vi "LIA-Simulator.vi"() -> ()   [LabVIEW 2018]
uses:
  <vilib>/addons/Digital Filter Design/_Objects.llb/DFD Multirate Filter Specification (Design).ctl
  <vilib>/addons/Digital Filter Design/_Objects.llb/DFD Filter Ripple Specification (Design).ctl
  <vilib>/Analysis/4window.llb/windowTd.ctl
  <vilib>/addons/Digital Filter Design/Analysis.llb/DFD Plot Freq Response (Linear-Spaced).vi
  <vilib>/addons/Digital Filter Design/Design.llb/DFD MRate Filter Design (Integer).vi
  <vilib>/addons/Digital Filter Design/Process.llb/DFD Filtering (Array).vi
  <vilib>/Analysis/2dsp.llb/Decimate (continuous, CDB).vi
  <vilib>/addons/Digital Filter Design/Multirate.llb/DFD MRate Filtering for Single Block (Array).vi
  <vilib>/measure/maspectr.llb/FFT Power Spectrum and PSD for 1 Chan (CDB).vi
  <vilib>/measure/maspectr.llb/FFT Power Spectrum and PSD for 1 Chan.vi
  <vilib>/measure/NI_MAPro.lvlib
  <vilib>/Analysis/NI_AALPro.lvlib
  <vilib>/addons/Digital Filter Design/NI_DigFilterLicensed.lvlib
  <vilib>/Analysis/NI_AALBase.lvlib
panel:
  in  "Iterations":i32=10
  out "FFT Gain":dbl
  out "Audio Depth":dbl format="%#_p"
  in  "Resolution":dbl=19.0 format="%#_13g"
  in  "Sampling Rate":dbl=1.0 format="%#_p"
  in  "Number Samples":i32=100000
  out "Error Out":errorcluster
  in  "Error In":errorcluster
  in  "Stop":bool
  in  "Tab Control 3":T1(tab)
  out "Noise vrms":dbl
  out "Noise (W|50ohms)":dbl
  out "k":dbl
  out "standard deviation":dbl format="%0.2p"
  out "mean":dbl format="%0.2p"
  out "standard deviation 2":dbl format="%0.2p"
  out "mean 2":dbl format="%0.2p"
  out "mean 3":dbl format="%0.2p"
  out "standard deviation 3":dbl format="%0.2p"
  in  "Tab Control 2":T2(tab)
  out "Waveform Graph 1":dbl[][](graph)
  out "Waveform Graph 3":cluster{"f0":dbl, "df":dbl, "magnitude":dbl[]}(graph)
  out "Waveform Graph 8":dbl[][](graph)
  out "Waveform Graph 7":cluster{"f0":dbl, "df":dbl, "magnitude":dbl[]}(graph)
  out "Waveform Graph 10":dbl[](graph)
  out "Waveform Graph 9":cluster{"f0":dbl, "df":dbl, "magnitude":dbl[]}(graph)
  out "Waveform Graph 12":dbl[](graph)
  out "Waveform Graph 11":cluster{"f0":dbl, "df":dbl, "magnitude":dbl[]}(graph)
  out "Waveform Graph 14":dbl[][](graph)
  out "Waveform Graph 13":cluster{"f0":dbl, "df":dbl, "magnitude":dbl[]}(graph)
  out "Waveform Graph 17":cluster{"f0":dbl, "df":dbl, "values":dbl[]}[](graph)
  out "Waveform Graph 16":dbl[](graph)
  out "Waveform Graph 15":cluster{"f0":dbl, "df":dbl, "magnitude":dbl[]}(graph)
  out "Waveform Graph 21":cluster{"f0":dbl, "df":dbl, "values":dbl[]}[](graph)
  out "Waveform Graph 23":dbl[](graph)
  out "Waveform Graph 22":cluster{"f0":dbl, "df":dbl, "magnitude":dbl[]}(graph)
  out "Waveform Graph 18":cluster{"f0":dbl, "df":dbl, "values":dbl[]}[](graph)
  out "Waveform Graph 20":dbl[](graph)
  out "Waveform Graph 19":cluster{"f0":dbl, "df":dbl, "magnitude":dbl[]}(graph)
  in  "Tab Control 1":T3(tab)
  in  "Oscillator Frequency":dbl=0.1 format="%#_p"
  in  "Oscillator Magnitude":dbl=1.0 format="%#_13g"
  in  "Signal Frequency":dbl=0.1 format="%#_p"
  in  "Signal Offset":cdb format="%#_13g"
  in  "Singal Amplitude":dbl=1.0 format="%#_13g"
  in  "Desired SNR (dB)":dbl format="%#_p"
  in  "low cutoff freq [Hz] 1":dbl=0.2
  in  "stopband atten [dB] 1":dbl=60.0 format="%.2f"
  in  "Decimation 1":i32=4
  in  "Decimation 2":i32=16
  in  "ripple specs":T4={"passband"=0.1, "stopband"=20.0, "dB/linear? (T: dB)"=TRUE}
  in  "freq specs [Hz]":T5={"fpass"=0.001, "fstop"=0.002}
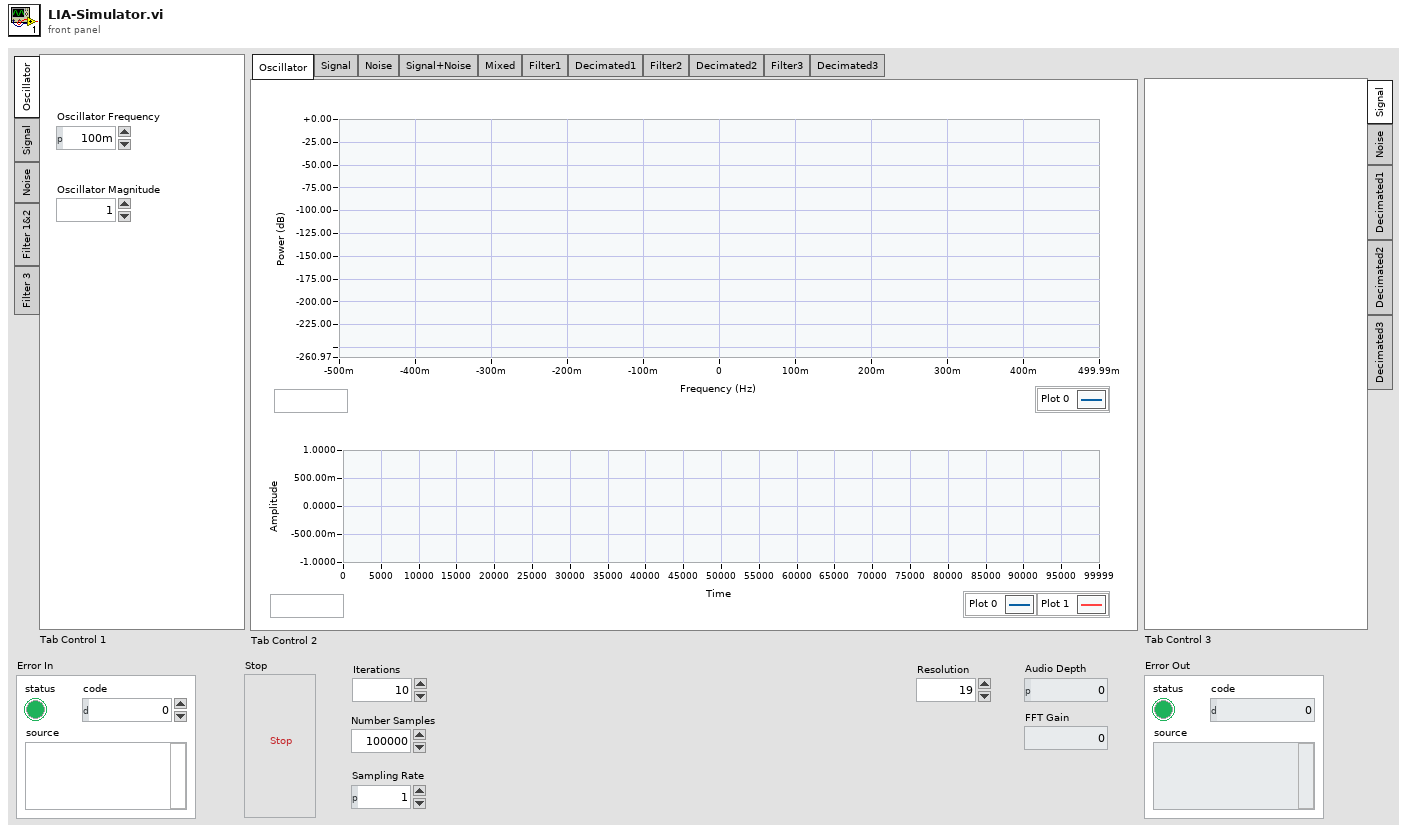
[diagram p1: front panel]
types:
  T1 = enum32{"Signal", "Noise", "Decimated1", "Decimated2", "Decimated3"}
  T2 = enum32{"Oscillator", "Signal", "Noise", "Signal+Noise", "Mixed", "Filter1", "Decimated1", "Filter2", "Decimated2", "Filter3", "Decimated3"}
  T3 = enum32{"Oscillator", "Signal", "Noise", "Filter 1&2", "Filter 3"}
  T4 = typedef "NI_DigFilterLicensed.lvlib/DFD Filter Ripple Specification (Design).ctl" = cluster{"passband":dbl, "stopband":dbl, "dB/linear? (T: dB)":bool}
  T5 = typedef "NI_DigFilterLicensed.lvlib/DFD Multirate Filter Specification (Design).ctl" = cluster{"fpass":dbl, "fstop":dbl}
  T6 = typedef "NI_DigFilterLicensed.lvlib/DFD Filter Obj.ctl" = cluster{"mSRate_Fs":dbl, "mSRate_Version":string, "mSRate_Comments":string, "mSRate_OrgCoef":T7, "mSRate_CurCoef":T7, "mSRate_Quantized?":bool, "mSRate_QCoef":T7, "mSRate_QSettings":T9[], "mSRate_Order":i32, "mSRate_Scaling":cluster{"mSRate_ScaleByPowerOf2?":bool, "mSRate_ScaleType":T11}}
  T7 = typedef "NI_DigFilterLicensed.lvlib/DFD Filter Coef.ctl" = cluster{"type":T8, "gain":dbl, "coef a (k)":dbl[], "coef b (v)":dbl[]}
  T8 = typedef "NI_DigFilterLicensed.lvlib/DFD Filter Structure Type Selector.ctl" = enum16{"Undefined", "FIR Direct Form", "FIR Direct Form Transposed", "FIR Symmetric", "FIR Antisymmetric", "IIR Direct Form I", "IIR Direct Form I Transposed", "IIR Direct Form II", "IIR Direct Form II Transposed", "IIR Cascaded Second Order Sections Form I", "IIR Cascaded Second Order Sections Form I Transposed", "IIR Cascaded Second Order Sections Form II", "IIR Cascaded Second Order Sections Form II Transposed", "Lattice Allpass (basic sections)", "Lattice Allpass (one multiplier sections)", "Lattice Allpass (normalized sections)", "Lattice AR (basic sections)", "Lattice AR (one multiplier sections)", "Lattice AR (normalized sections)", "Lattice MA (minimum phase)", "Lattice MA (maximum phase)", "Lattice ARMA (basic sections)", "Lattice ARMA (one multiplier sections)", "Lattice ARMA (normalized sections)"}
  T9 = typedef "NI_DigFilterLicensed.lvlib/dfd_Internal Quantization Settings.ctl" = cluster{"source":T10, "wl":i16, "iwl":i16, "overflow mode":enum16{"Saturation", "Wrap"}, "rounding mode":enum16{"Nearest", "Truncation"}, "signed?":bool}
  T10 = typedef "NI_DigFilterLicensed.lvlib/dfd_Internal Quantization Srcs.ctl" = u16
  T11 = typedef "NI_DigFilterLicensed.lvlib/DFD Coef Norm Type.ctl" = enum16{"No Norm", "Time Domain 1-Norm", "Time Domain 2-Norm", "Time Domain Inf-Norm"}
  T12 = typedef "NI_DigFilterLicensed.lvlib/DFD Multirate Filter Obj.ctl" = cluster{"mMRate_Structure":enum16{"CIC", "FIR", "IIR", "Lattice"}, "mMRate_Mode":T13, "mMRate_Factor":i32, "mMRate_FIRParams":cluster{"mMRate_FIR_H":dbl[], "mMRate_FIR_IsNyquist?":bool, "mMRate_FIR_IsSymmetric?":bool}, "mMRate_CICParams":cluster{"mMRate_CIC_#Stage":i32, "mMRate_CIC_Lag":i32, "mMRate_CIC_Type":enum16{"Lowpass", "Highpass"}}, "mMRate_Order":i32, "mMRate_Version":string, "mMRate_Comments":string, "mMRate_RationalFactor":cluster{"mMRate_L":i32, "mMRate_M":i32}, "mMRate_Fs":dbl, "mMRate_Quantized?":bool, "mMRate_QFilterGain":dbl, "mMRate_CoefWl":i16, "mMRate_Scaling":cluster{"mMRate_ScaleByPowerOf2?":bool, "mMRate_ScaleType":T11}, "mMRate_InputWl":i16, "mMRate_OutputWl":i16, "mMRate_OutputMode":T14, "mMRate_MultMode":T15, "mMRate_BitPruning":bool, "mMRate_GainWl":i16, "mMRate_OutputFwl":i16, "mMRate_SumIwl":i16, "mMRate_InputIwl ":i16, "mMRate_SumWl":i16, "mMRate_CoefIwl":i16}
  T13 = typedef "NI_DigFilterLicensed.lvlib/DFD Multirate Mode.ctl" = i16
  T14 = typedef "NI_DigFilterLicensed.lvlib/DFD Round-off Mode.ctl" = enum16{"Nearest", "Truncation"}
  T15 = typedef "NI_DigFilterLicensed.lvlib/DFD FXP MRate Multiply Mode.ctl" = enum16{"Truncated", "Full"}
  T16 = cluster{"averaging mode":enum16{"No averaging", "Vector averaging", "RMS averaging", "Peak hold"}, "weighting mode":enum16{"Linear", "Exponential"}, "number of averages":u32}
  T17 = typedef "NI_AALPro.lvlib/windowTd.ctl" = u32
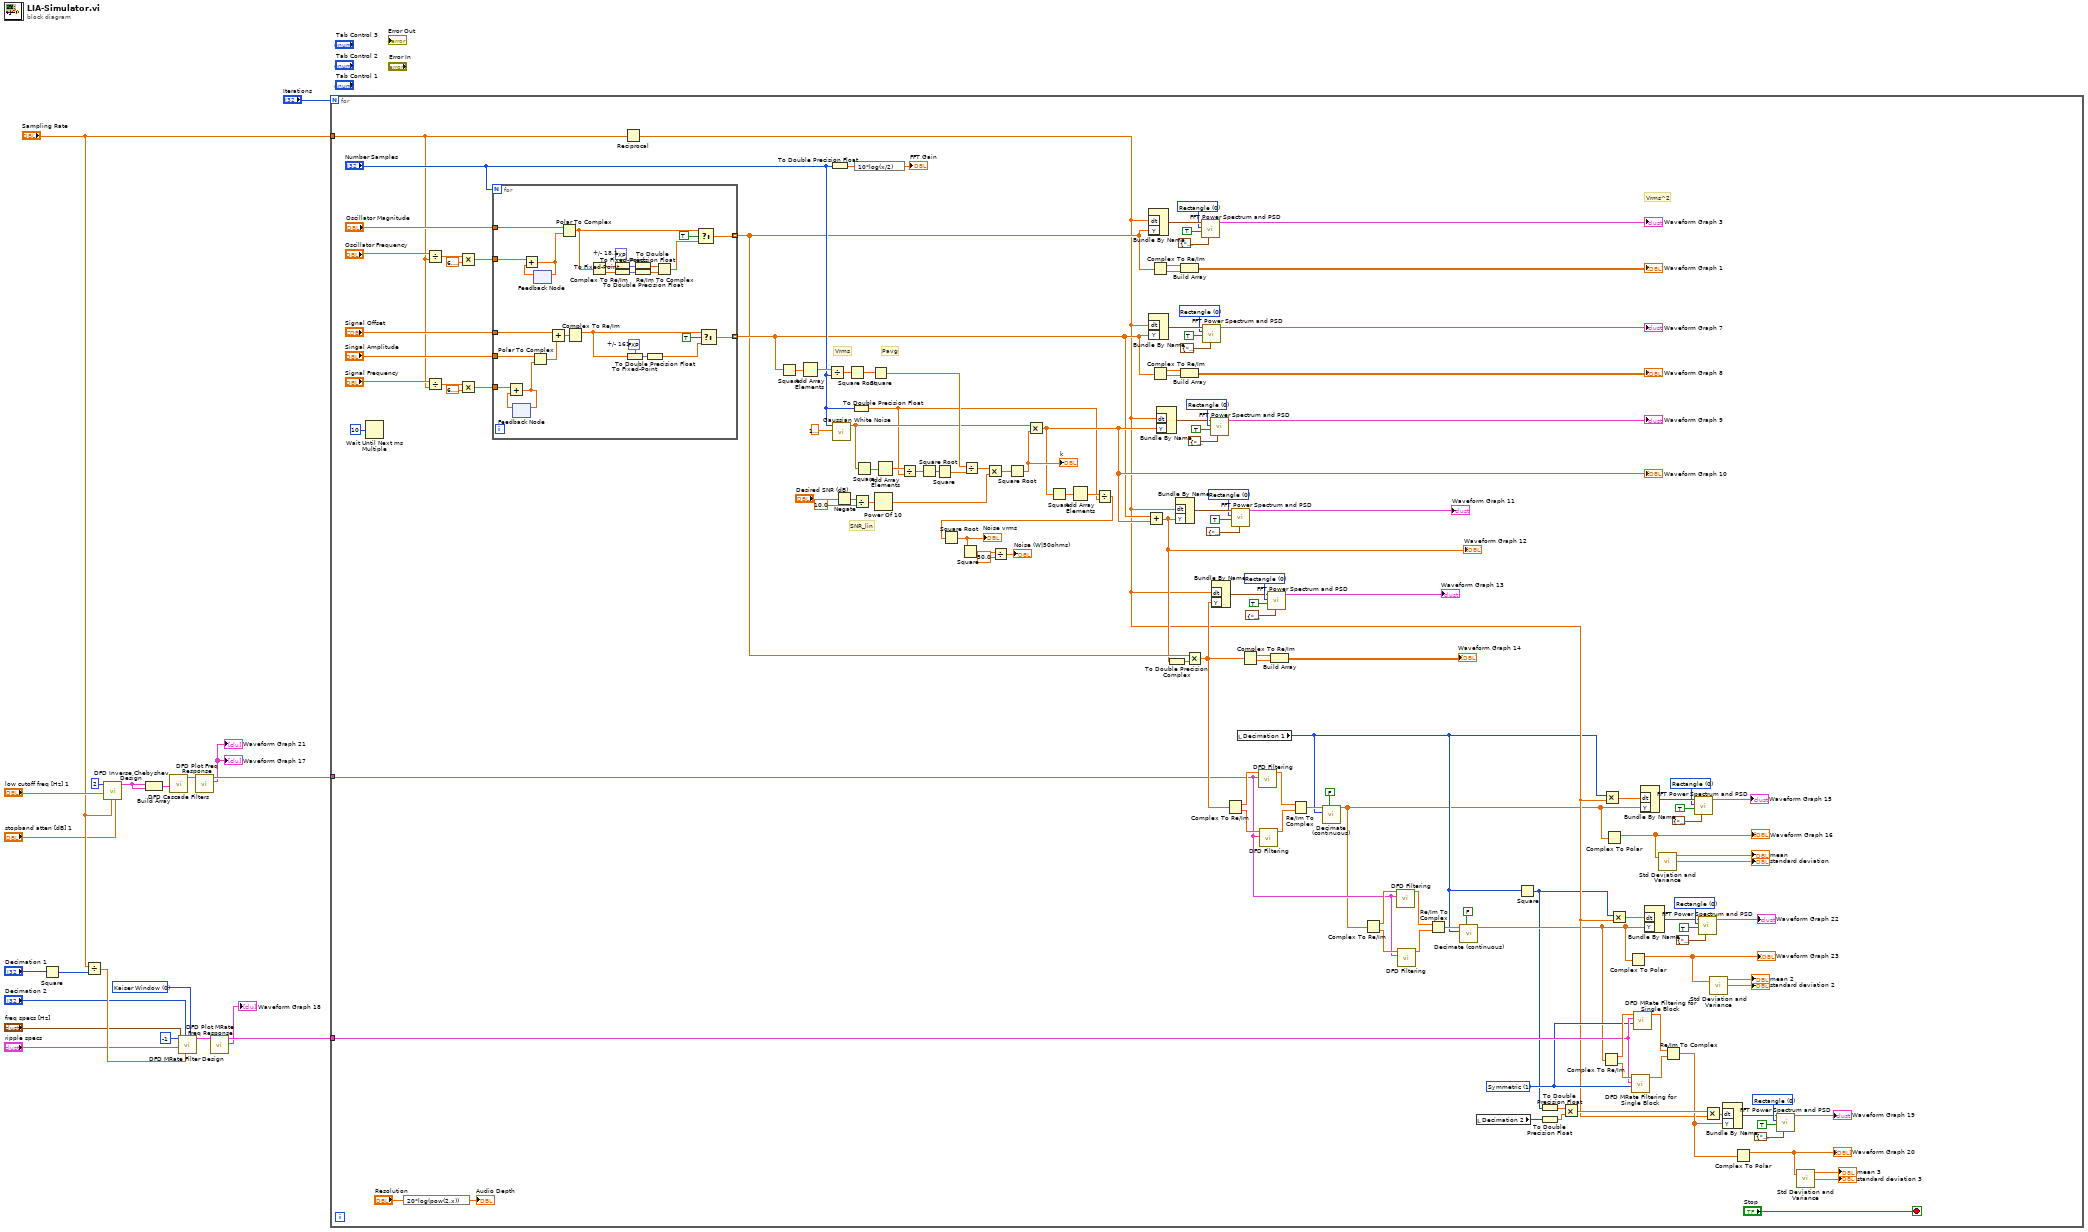
[diagram p0: block diagram]
diagram:
  w5 = u16 0 items=["Kaiser Window", "Dolph-Chebyshev Window", "Equi-Ripple"] ("method")
  n1 = Square(x="Decimation 1") -> (x^2=w1:i32)
  n2 = Divide(x="Sampling Rate", y=w1) -> (x/y=w10:dbl)
  n3 = call <vilib>:"DFD Inverse Chebyshev Design.vi"("stopband atten [dB]"="stopband atten [dB] 1", "fs [Hz]"="Sampling Rate", "low cutoff freq [Hz]"="low cutoff freq [Hz] 1", "order"=2) -> ("filter out"=w15:T6)  [unwired: 6 in, 1 out]
  n4 = Build Array(w15, w15) -> (w20:T6[])
  n5 = call <vilib>:"DFD Cascade Filters.vi"("filters in"=w20) -> ("filter out"=w16:T6)  [unwired: 9 in, 1 out]
  n6 = call-poly <vilib>:"DFD MRate Filter Design.vi"("method"=w5, "fs in [Hz]"=w10, "factor"="Decimation 2", "ripple specs"="ripple specs", "freq specs [Hz]"="freq specs [Hz]", "order"=-1) -> ("multirate filter out"=w9:T12)  [unwired: 4 in, 1 out]
  n7 = call-poly <vilib>:"DFD Plot Freq Response.vi"("filter in"=w16) -> ("magnitude response"=→"Waveform Graph 17" →"Waveform Graph 21":cluster{"f0":dbl, "df":dbl, "values":dbl[]}[], "filter out"=w11:T6)  [unwired: 7 in, 2 out]
  n8 = call <vilib>:"DFD Plot MRate Freq Response.vi"("multirate filter in"=w9) -> ("magnitude response"=→"Waveform Graph 18":cluster{"f0":dbl, "df":dbl, "values":dbl[]}[], "multirate filter out"=w12:T12)  [unwired: 7 in, 2 out]
  n9 = for {
    N: "Iterations" -> [_]
    tunnel: "Sampling Rate" -> [w74]
    tunnel: w12 -> [w50]
    tunnel: w11 -> [w37]
    stop <- "Stop" stop-if-true
    w35 = T17 0 items=["Rectangle"=0, "Hanning"=1, "Hamming"=2, "Blackman-Harris"=3, "Exact Blackman"=4, "Blackman"=5, "Flat Top"=6, "4 Term B-Harris "=7, "7 Term B-Harris"=8, "Low Sidelobe"=9, "Blackman Nuttall"=11, "Triangle"=30, "Bartlett-Hanning"=31, "Bohman"=32, "Parzen"=33, "Welch"=34, "Kaiser"=60, "Dolph-Chebyshev"=61, "Gaussian"=62] ("window")
    w46 = u16 1 items=["Zero padding", "Symmetric", "Periodic"] ("extension type")
    w62 = T17 0 items=["Rectangle"=0, "Hanning"=1, "Hamming"=2, "Blackman-Harris"=3, "Exact Blackman"=4, "Blackman"=5, "Flat Top"=6, "4 Term B-Harris "=7, "7 Term B-Harris"=8, "Low Sidelobe"=9, "Blackman Nuttall"=11, "Triangle"=30, "Bartlett-Hanning"=31, "Bohman"=32, "Parzen"=33, "Welch"=34, "Kaiser"=60, "Dolph-Chebyshev"=61, "Gaussian"=62] ("window")
    w79 = T17 0 items=["Rectangle"=0, "Hanning"=1, "Hamming"=2, "Blackman-Harris"=3, "Exact Blackman"=4, "Blackman"=5, "Flat Top"=6, "4 Term B-Harris "=7, "7 Term B-Harris"=8, "Low Sidelobe"=9, "Blackman Nuttall"=11, "Triangle"=30, "Bartlett-Hanning"=31, "Bohman"=32, "Parzen"=33, "Welch"=34, "Kaiser"=60, "Dolph-Chebyshev"=61, "Gaussian"=62] ("window")
    w90 = T17 0 items=["Rectangle"=0, "Hanning"=1, "Hamming"=2, "Blackman-Harris"=3, "Exact Blackman"=4, "Blackman"=5, "Flat Top"=6, "4 Term B-Harris "=7, "7 Term B-Harris"=8, "Low Sidelobe"=9, "Blackman Nuttall"=11, "Triangle"=30, "Bartlett-Hanning"=31, "Bohman"=32, "Parzen"=33, "Welch"=34, "Kaiser"=60, "Dolph-Chebyshev"=61, "Gaussian"=62] ("window")
    w100 = T17 0 items=["Rectangle"=0, "Hanning"=1, "Hamming"=2, "Blackman-Harris"=3, "Exact Blackman"=4, "Blackman"=5, "Flat Top"=6, "4 Term B-Harris "=7, "7 Term B-Harris"=8, "Low Sidelobe"=9, "Blackman Nuttall"=11, "Triangle"=30, "Bartlett-Hanning"=31, "Bohman"=32, "Parzen"=33, "Welch"=34, "Kaiser"=60, "Dolph-Chebyshev"=61, "Gaussian"=62] ("window")
    w140 = T17 0 items=["Rectangle"=0, "Hanning"=1, "Hamming"=2, "Blackman-Harris"=3, "Exact Blackman"=4, "Blackman"=5, "Flat Top"=6, "4 Term B-Harris "=7, "7 Term B-Harris"=8, "Low Sidelobe"=9, "Blackman Nuttall"=11, "Triangle"=30, "Bartlett-Hanning"=31, "Bohman"=32, "Parzen"=33, "Welch"=34, "Kaiser"=60, "Dolph-Chebyshev"=61, "Gaussian"=62] ("window")
    w144 = T17 0 items=["Rectangle"=0, "Hanning"=1, "Hamming"=2, "Blackman-Harris"=3, "Exact Blackman"=4, "Blackman"=5, "Flat Top"=6, "4 Term B-Harris "=7, "7 Term B-Harris"=8, "Low Sidelobe"=9, "Blackman Nuttall"=11, "Triangle"=30, "Bartlett-Hanning"=31, "Bohman"=32, "Parzen"=33, "Welch"=34, "Kaiser"=60, "Dolph-Chebyshev"=61, "Gaussian"=62] ("window")
    w152 = T17 0 items=["Rectangle"=0, "Hanning"=1, "Hamming"=2, "Blackman-Harris"=3, "Exact Blackman"=4, "Blackman"=5, "Flat Top"=6, "4 Term B-Harris "=7, "7 Term B-Harris"=8, "Low Sidelobe"=9, "Blackman Nuttall"=11, "Triangle"=30, "Bartlett-Hanning"=31, "Bohman"=32, "Parzen"=33, "Welch"=34, "Kaiser"=60, "Dolph-Chebyshev"=61, "Gaussian"=62] ("window")
    # "SNR_lin"
    # "Pavg"
    # "Vrms"
    # "Vrms^2"
    n10 = Wait Until Next ms Multiple(millisecond multiple=u32 10) -> ()  [unwired: 1 out]
    n11 = expression code="20*log(pow(2,x))"("Resolution") -> (→"Audio Depth":dbl)
    n12 = Divide(x="Oscillator Frequency", y=w74) -> (x/y=w136:dbl)
    n13 = Divide(x="Signal Frequency", y=w74) -> (x/y=w162:dbl)
    n14 = Multiply(x=w136, y=6.283185307179586) -> (x*y=w133:dbl)
    n15 = Multiply(x=w162, y=6.283185307179586) -> (x*y=w161:dbl)
    n16 = for {
      N: "Number Samples" -> [_]
      tunnel: w161 -> [w188]
      tunnel: "Singal Amplitude" -> [w191]
      tunnel: "Signal Offset" -> [w190]
      tunnel: [w174] -> w92 mode=indexing
      tunnel: [w168] -> w94 mode=indexing
      tunnel: w133 -> [w179]
      tunnel: "Oscillator Magnitude" -> [w177]
      w169 = fxp<+/-,16,1> 0.0  # +/- 161
      w184 = fxp<+/-,18,1> 0.0  # +/- 18,1
      n17 = feedback #1() -> (w192:dbl)  [unwired: 1 in]
      n18 = Add(x=w188, y=w192) -> (x+y=w187:dbl)
      n19 = feedback-in #1(w187) -> ()
      n20 = Polar To Complex(1:w187, 2:w191) -> (0:w189:cdb)
      n21 = feedback #2() -> (w178:dbl)  [unwired: 1 in]
      n22 = Add(x=w179, y=w178) -> (x+y=w176:dbl)
      n23 = feedback-in #2(w176) -> ()
      n24 = Add(x=w190, y=w189) -> (x+y=w166:cdb)
      n25 = Polar To Complex(1:w176, 2:w177) -> (0:w175:cdb)
      n26 = Complex To Re/Im(x + iy=w166) -> (x=w165:dbl)  [unwired: 1 out]
      n27 = Complex To Re/Im(x + iy=w175) -> (x=w186:dbl, y=w185:dbl)
      n28 = To Fixed-Point(fixed-point type=w184, number=w186) -> (fixed-point=w183:fxp<+/-,18,1>)
      n29 = To Fixed-Point(fixed-point type=w184, number=w185) -> (fixed-point=w182:fxp<+/-,18,1>)
      n30 = To Fixed-Point(fixed-point type=w169, number=w165) -> (fixed-point=w170:fxp<+/-,16,1>)
      n31 = To Double Precision Float(number=w183) -> (double precision float=w181:dbl)
      n32 = To Double Precision Float(number=w182) -> (double precision float=w180:dbl)
      n33 = To Double Precision Float(number=w170) -> (double precision float=w167:dbl)
      n34 = Re/Im To Complex(1:w180, 2:w181) -> (0:w173:cdb)
      n35 = Select(t=w175, s=TRUE, f=w173) -> (s? t:f=w174:cdb)
      n36 = Select(t=w165, s=TRUE, f=w167) -> (s? t:f=w168:dbl)
    }
    n37 = Reciprocal(x=w74) -> (1/x=w31:dbl)
    n38 = Square(x=w94) -> (x^2=w131:dbl[])
    n39 = Add Array Elements(numeric array=w131) -> (sum=w130:dbl)
    n40 = Divide(x=w130, y="Number Samples") -> (x/y=w129:dbl)
    n41 = To Double Precision Float(number="Number Samples") -> (double precision float=w96:dbl)
    n42 = call <vilib>:"Gaussian White Noise.vi"("standard deviation"=1.0000000000000002, "samples"="Number Samples") -> ("Gaussian noise pattern"=w113:dbl[])  [unwired: 8 in, 1 out]
    n43 = Negate(x="Desired SNR (dB)") -> (-x=w116:dbl)
    n44 = Square Root(x=w129) -> (sqrt(x)=w128:dbl)
    n45 = To Double Precision Float(number="Number Samples") -> (double precision float=w83:dbl)
    n46 = Divide(x=w116, y=10.0) -> (x/y=w124:dbl)
    n47 = expression code="10*log(x/2)"(w96) -> (→"FFT Gain":dbl)
    n48 = Square(x=w113) -> (x^2=w120:dbl[])
    n49 = Square(x=w128) -> (x^2=w119:dbl)
    n50 = Power Of 10(x=w124) -> (10^x=w115:dbl)
    n51 = Add Array Elements(numeric array=w120) -> (sum=w121:dbl)
    n52 = Divide(x=w121, y=w83) -> (x/y=w122:dbl)
    n53 = Square Root(x=w122) -> (sqrt(x)=w123:dbl)
    n54 = Square(x=w123) -> (x^2=w118:dbl)
    n55 = Divide(x=w119, y=w118) -> (x/y=w117:dbl)
    n56 = Multiply(x=w117, y=w115) -> (x*y=w114:dbl)
    n57 = Square Root(x=w114) -> (sqrt(x)=w112:dbl)
    "k" <- w112
    n58 = Multiply(x=w113, y=w112) -> (x*y=w99:dbl[])
    "Waveform Graph 10" <- w99
    n59 = Square(x=w99) -> (x^2=w111:dbl[])
    n60 = Add Array Elements(numeric array=w111) -> (sum=w110:dbl)
    n61 = Divide(x=w110, y=w83) -> (x/y=w109:dbl)
    n62 = Square Root(x=w109) -> (sqrt(x)=w108:dbl)
    "Noise vrms" <- w108
    n63 = Square(x=w108) -> (x^2=w107:dbl)
    n64 = Divide(x=w107, y=50.0) -> (x/y=→"Noise (W|50ohms)":dbl)
    n65 = Add(x=w94, y=w99) -> (x+y=w91:dbl[])
    "Waveform Graph 12" <- w91
    n66 = Bundle By Name("dt"=w31, "Y"=w92) -> (w155:waveform(cdb))  [unwired: 1 in]
    n67 = Bundle By Name("dt"=w31, "Y"=w94) -> (w147:waveform(dbl))  [unwired: 1 in]
    n68 = Complex To Re/Im(x + iy=w92) -> (x=w150:dbl[], y=w149:dbl[])
    n69 = Complex To Re/Im(x + iy=w94) -> (x=w143:dbl[], y=w142:dbl[])
    n70 = Bundle By Name("dt"=w31, "Y"=w99) -> (w137:waveform(dbl))  [unwired: 1 in]
    n71 = To Double Precision Complex(1:w91) -> (0:w77:cdb[])
    n72 = Bundle By Name("dt"=w31, "Y"=w91) -> (w103:waveform(dbl))  [unwired: 1 in]
    n73 = Build Array(w150, w149) -> (→"Waveform Graph 1":dbl[][])
    n74 = Build Array(w143, w142) -> (→"Waveform Graph 8":dbl[][])
    n75 = Multiply(x=w92, y=w77) -> (x*y=w76:cdb[])
    n76 = call-poly <vilib>:"FFT Power Spectrum and PSD.vi"("averaging parameters"=T16 {"averaging mode"=enum."No averaging", "weighting mode"=enum."Exponential", "number of averages"=10}, "dB On (F)"=TRUE, "window"=w152, "time signal"=w155) -> ("Power Spectrum / PSD"=→"Waveform Graph 3":cluster{"f0":dbl, "df":dbl, "magnitude":dbl[]})  [unwired: 4 in, 3 out]
    n77 = call-poly <vilib>:"FFT Power Spectrum and PSD.vi"("averaging parameters"=T16 {"averaging mode"=enum."RMS averaging", "weighting mode"=enum."Exponential", "number of averages"=10}, "dB On (F)"=TRUE, "window"=w144, "time signal"=w147) -> ("Power Spectrum / PSD"=→"Waveform Graph 7":cluster{"f0":dbl, "df":dbl, "magnitude":dbl[]})  [unwired: 4 in, 3 out]
    n78 = call-poly <vilib>:"FFT Power Spectrum and PSD.vi"("averaging parameters"=T16 {"averaging mode"=enum."RMS averaging", "weighting mode"=enum."Exponential", "number of averages"=10}, "dB On (F)"=TRUE, "window"=w140, "time signal"=w137) -> ("Power Spectrum / PSD"=→"Waveform Graph 9":cluster{"f0":dbl, "df":dbl, "magnitude":dbl[]})  [unwired: 4 in, 3 out]
    n79 = Bundle By Name("dt"=w31, "Y"=w76) -> (w87:waveform(cdb))  [unwired: 1 in]
    n80 = Complex To Re/Im(x + iy=w76) -> (x=w69:dbl[], y=w68:dbl[])
    n81 = call-poly <vilib>:"FFT Power Spectrum and PSD.vi"("averaging parameters"=T16 {"averaging mode"=enum."RMS averaging", "weighting mode"=enum."Exponential", "number of averages"=10}, "dB On (F)"=TRUE, "window"=w100, "time signal"=w103) -> ("Power Spectrum / PSD"=→"Waveform Graph 11":cluster{"f0":dbl, "df":dbl, "magnitude":dbl[]})  [unwired: 4 in, 3 out]
    n82 = local read "Decimation 1"() -> (w30:i32)
    n83 = Complex To Re/Im(x + iy=w76) -> (x=w85:dbl[], y=w86:dbl[])
    n84 = call-poly <vilib>:"DFD Filtering.vi"("filter"=w37, "signal in"=w69) -> ("signal out"=w67:dbl[])  [unwired: 8 in, 1 out]
    n85 = call-poly <vilib>:"DFD Filtering.vi"("filter"=w37, "signal in"=w68) -> ("signal out"=w66:dbl[])  [unwired: 8 in, 1 out]
    n86 = call-poly <vilib>:"FFT Power Spectrum and PSD.vi"("averaging parameters"=T16 {"averaging mode"=enum."RMS averaging", "weighting mode"=enum."Exponential", "number of averages"=10}, "dB On (F)"=TRUE, "window"=w90, "time signal"=w87) -> ("Power Spectrum / PSD"=→"Waveform Graph 13":cluster{"f0":dbl, "df":dbl, "magnitude":dbl[]})  [unwired: 4 in, 3 out]
    n87 = Build Array(w85, w86) -> (→"Waveform Graph 14":dbl[][])
    n88 = Re/Im To Complex(1:w66, 2:w67) -> (0:w65:cdb[])
    n89 = call-poly <vilib>:"Decimate (continuous).vi"("reset"=FALSE, "decimating factor"=w30, "X"=w65) -> ("Decimated Array"=w28:cdb[])  [unwired: 7 in, 1 out]
    n90 = Complex To Re/Im(x + iy=w28) -> (x=w38:dbl[], y=w39:dbl[])
    n91 = call-poly <vilib>:"DFD Filtering.vi"("filter"=w37, "signal in"=w38) -> ("signal out"=w40:dbl[])  [unwired: 8 in, 1 out]
    n92 = call-poly <vilib>:"DFD Filtering.vi"("filter"=w37, "signal in"=w39) -> ("signal out"=w41:dbl[])  [unwired: 8 in, 1 out]
    n93 = Re/Im To Complex(1:w41, 2:w40) -> (0:w42:cdb[])
    n94 = call-poly <vilib>:"Decimate (continuous).vi"("reset"=FALSE, "decimating factor"=w30, "X"=w42) -> ("Decimated Array"=w26:cdb[])  [unwired: 7 in, 1 out]
    n95 = local read "Decimation 2"() -> (w49:i32)
    n96 = Square(x=w30) -> (x^2=w25:i32)
    n97 = To Double Precision Float(number=w25) -> (double precision float=w44:dbl)
    n98 = To Double Precision Float(number=w49) -> (double precision float=w45:dbl)
    n99 = Multiply(x=w44, y=w45) -> (x*y=w55:dbl)
    n100 = Complex To Re/Im(x + iy=w26) -> (x=w54:dbl[], y=w52:dbl[])
    n101 = Multiply(x=w30, y=w31) -> (x*y=w64:dbl)
    n102 = Complex To Polar(r * e^(i*theta)=w28) -> (r=w72:dbl[])  [unwired: 1 out]
    "Waveform Graph 16" <- w72
    n103 = Multiply(x=w25, y=w31) -> (x*y=w36:dbl)
    n104 = Complex To Polar(r * e^(i*theta)=w26) -> (r=w27:dbl[])  [unwired: 1 out]
    "Waveform Graph 23" <- w27
    n105 = call-poly <vilib>:"DFD MRate Filtering for Single Block.vi"("extension type"=w46, "multirate filter"=w50, "signal in"=w52) -> ("signal out"=w51:dbl[])  [unwired: 7 in, 1 out]
    n106 = call-poly <vilib>:"DFD MRate Filtering for Single Block.vi"("extension type"=w46, "multirate filter"=w50, "signal in"=w54) -> ("signal out"=w53:dbl[])  [unwired: 7 in, 1 out]
    n107 = Bundle By Name("dt"=w64, "Y"=w28) -> (w82:waveform(cdb))  [unwired: 1 in]
    n108 = Bundle By Name("dt"=w36, "Y"=w26) -> (w32:waveform(cdb))  [unwired: 1 in]
    n109 = call <vilib>:"Std Deviation and Variance.vi"("X"=w72) -> ("mean"=→"mean":dbl, "standard deviation"=→"standard deviation":dbl)  [unwired: 1 in, 1 out]
    n110 = Re/Im To Complex(1:w51, 2:w53) -> (0:w48:cdb[])
    n111 = call-poly <vilib>:"FFT Power Spectrum and PSD.vi"("averaging parameters"=T16 {"averaging mode"=enum."RMS averaging", "weighting mode"=enum."Exponential", "number of averages"=10}, "dB On (F)"=TRUE, "window"=w79, "time signal"=w82) -> ("Power Spectrum / PSD"=→"Waveform Graph 15":cluster{"f0":dbl, "df":dbl, "magnitude":dbl[]})  [unwired: 4 in, 3 out]
    n112 = call-poly <vilib>:"FFT Power Spectrum and PSD.vi"("averaging parameters"=T16 {"averaging mode"=enum."RMS averaging", "weighting mode"=enum."Exponential", "number of averages"=10}, "dB On (F)"=TRUE, "window"=w35, "time signal"=w32) -> ("Power Spectrum / PSD"=→"Waveform Graph 22":cluster{"f0":dbl, "df":dbl, "magnitude":dbl[]})  [unwired: 4 in, 3 out]
    n113 = Multiply(x=w55, y=w31) -> (x*y=w63:dbl)
    n114 = call <vilib>:"Std Deviation and Variance.vi"("X"=w27) -> ("mean"=→"mean 2":dbl, "standard deviation"=→"standard deviation 2":dbl)  [unwired: 1 in, 1 out]
    n115 = Bundle By Name("dt"=w63, "Y"=w48) -> (w59:waveform(cdb))  [unwired: 1 in]
    n116 = Complex To Polar(r * e^(i*theta)=w48) -> (r=w22:dbl[])  [unwired: 1 out]
    "Waveform Graph 20" <- w22
    n117 = call-poly <vilib>:"FFT Power Spectrum and PSD.vi"("averaging parameters"=T16 {"averaging mode"=enum."RMS averaging", "weighting mode"=enum."Exponential", "number of averages"=10}, "dB On (F)"=TRUE, "window"=w62, "time signal"=w59) -> ("Power Spectrum / PSD"=→"Waveform Graph 19":cluster{"f0":dbl, "df":dbl, "magnitude":dbl[]})  [unwired: 4 in, 3 out]
    n118 = call <vilib>:"Std Deviation and Variance.vi"("X"=w22) -> ("mean"=→"mean 3":dbl, "standard deviation"=→"standard deviation 3":dbl)  [unwired: 1 in, 1 out]
  }
